vi "Read_IMU.vi"(6 "error in (no error) 2":errorcluster, 8 "IMU_SS":T1, 9 "SPI Ref In":T8={"myRIO Reference"={"myRIO Model"=enum."Unknown", "myRIO Hardware Reference"={"Generic FPGA Reference"=refnum, "Allow multiple opens"=FALSE}}, "SPI Channels Enum"=enum."Not Connected", "SPI Configuration"={"Frequency [Hz]"=0.0, "Clock Phase"=enum."Leading", "Clock Polarity"=enum."Low", "Data Direction"=enum."Most significant bit first", "Frame Length"=8}} {"SPI Configuration"."Frame Length" min=1 max=16}) -> (0 "error out":errorcluster, 1 "Roll":dbl, 2 "Yaw":dbl, 3 "Pitch":dbl)   [LabVIEW 2018]
uses:
  <vilib>/myRIO/Instrument Drivers/Onboard IO/SPI/typedefs/SPI Reference.ctl
  <vilib>/myRIO/Common/Instrument Driver Framework/Utilities/typedefs/myRIO Generic Hardware Reference.ctl
  <vilib>/myRIO/Common/Instrument Driver Framework/Utilities/typedefs/Hardware Version Enum.ctl
  <vilib>/myRIO/Common/Instrument Driver Framework/Utilities/typedefs/myRIO v1.0 Reference.ctl
  <vilib>/myRIO/Common/Instrument Driver Framework/Utilities/typedefs/Generic FPGA Reference.ctl
  <vilib>/myRIO/Common/Instrument Driver Framework/myRIO v1.0/SPI/typedefs/SPI Channels Enum.ctl
  <vilib>/myRIO/Instrument Drivers/Onboard IO/SPI/typedefs/SPI Configuration.ctl
  <vilib>/myRIO/Common/Instrument Driver Framework/myRIO v1.0/SPI/typedefs/SPI Clock Phase.ctl
  <vilib>/myRIO/Common/Instrument Driver Framework/myRIO v1.0/SPI/typedefs/SPI Clock Polarity.ctl
  <vilib>/myRIO/Common/Instrument Driver Framework/myRIO v1.0/SPI/typedefs/SPI Data Direction.ctl
  <vilib>/myRIO/Common/Instrument Driver Framework/myRIO v1.0/SPI/typedefs/SPI Frame Length.ctl
  <vilib>/myRIO/Instrument Drivers/Onboard IO/DIO/typedefs/DIO Reference.ctl
  <vilib>/myRIO/Common/Instrument Driver Framework/myRIO v1.0/DIO/typedefs/DIO Channels List.ctl
  <vilib>/myRIO/Common/Instrument Driver Framework/myRIO v1.0/DIO/typedefs/DIO Channels Enum.ctl
  <vilib>/Utility/error.llb/Error Cluster From Error Code.vi
  <vilib>/myRIO/Common/Instrument Driver Framework/myRIO v1.0/DIO/vis/myRIO v1.0 Write DIO.vi
  <vilib>/myRIO/Common/Instrument Driver Framework/myRIO v1.0/SPI/vis/myRIO v1.0 Write Read SPI.vi
  <vilib>/myRIO/Instrument Drivers/Onboard IO/SPI/SPI.lvlib
  <vilib>/myRIO/Instrument Drivers/Onboard IO/DIO/DIO.lvlib
panel:
  out "subarray":u16[](array[numeric])
  out "IMU":sgl[](array[numeric])
  out "IMU_SS":T1
  out "SPI Ref Out":T8={"myRIO Reference"={"myRIO Model"=enum."Unknown", "myRIO Hardware Reference"={"Generic FPGA Reference"=refnum, "Allow multiple opens"=FALSE}}, "SPI Channels Enum"=enum."Not Connected", "SPI Configuration"={"Frequency [Hz]"=0.0, "Clock Phase"=enum."Leading", "Clock Polarity"=enum."Low", "Data Direction"=enum."Most significant bit first", "Frame Length"=8}} {"SPI Configuration"."Frame Length" min=1 max=16}
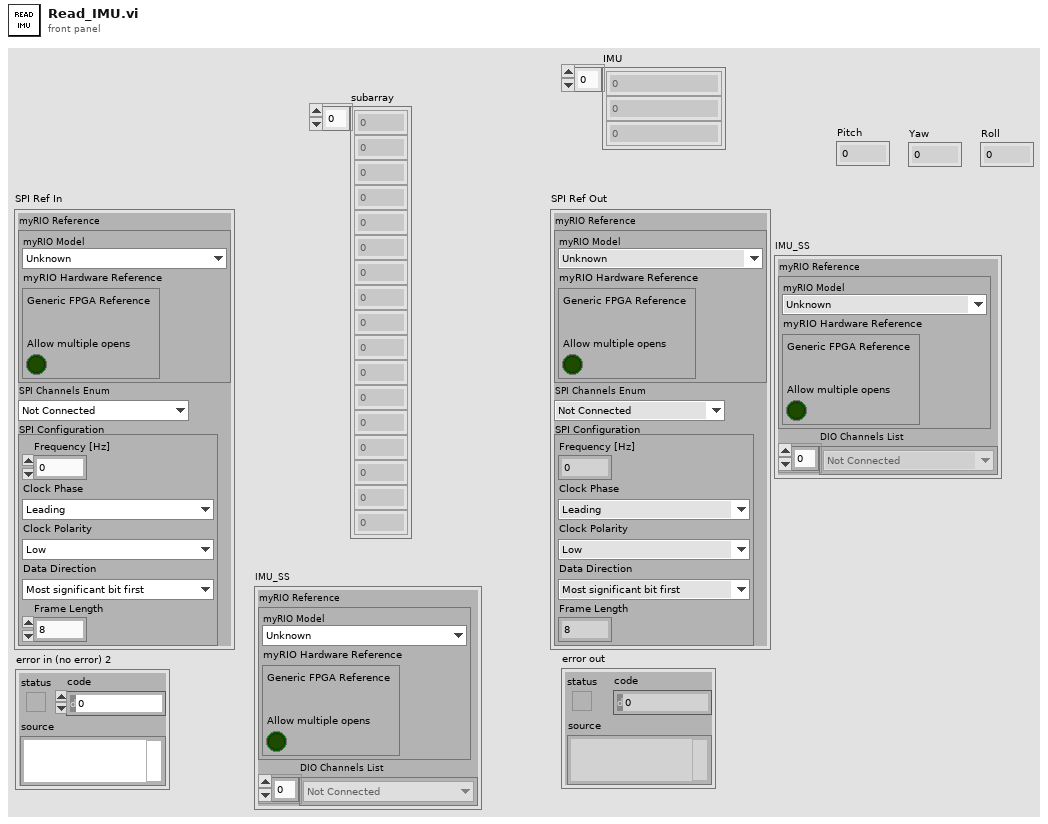
[diagram p1: front panel]
types:
  T1 = typedef "DIO.lvlib/DIO Reference.ctl" = cluster{"myRIO Reference":T2, "DIO Channels List":T6}
  T2 = typedef "myRIO Generic Hardware Reference.ctl" = cluster{"myRIO Model":T3, "myRIO Hardware Reference":T4}
  T3 = typedef "Hardware Version Enum.ctl" = enum16{"Unknown", "myRIO-1900", "myRIO-1950", "roboRIO", "NI ELVIS RIO CM", "ELVIS III"}
  T4 = typedef "myRIO v1.0 Reference.ctl" = cluster{"Generic FPGA Reference":T5, "Allow multiple opens":bool}
  T5 = typedef "Generic FPGA Reference.ctl" = refnum<k20>
  T6 = typedef "DIO Channels List.ctl" = T7[]
  T7 = typedef "DIO Channels Enum.ctl" = enum16{"Not Connected", "C/DIO0", "C/DIO1", "C/DIO2", "C/DIO3", "C/DIO4", "C/DIO5", "C/DIO6", "C/DIO7", "A/DIO0", "A/DIO1", "A/DIO2", "A/DIO3", "A/DIO4", "A/DIO5", "A/DIO6", "A/DIO7", "A/DIO8", "A/DIO9", "A/DIO10", "A/DIO11", "A/DIO12", "A/DIO13", "A/DIO14", "A/DIO15", "A/DIO16", "A/DIO17", "A/DIO18", "A/DIO19", "B/DIO0", "B/DIO1", "B/DIO2", "B/DIO3", "B/DIO4", "B/DIO5", "B/DIO6", "B/DIO7", "B/DIO8", "B/DIO9", "B/DIO10", "B/DIO11", "B/DIO12", "B/DIO13", "B/DIO14", "B/DIO15", "B/DIO16", "B/DIO17", "B/DIO18", "B/DIO19", "LED0", "LED1", "LED2", "LED3", "Button0", "DIO/DIO0", "DIO/DIO1", "DIO/DIO2", "DIO/DIO3", "DIO/DIO4", "DIO/DIO5", "DIO/DIO6", "DIO/DIO7", "DIO/DIO8", "DIO/DIO9", "SPI/CS0", "SPI/CS1", "SPI/CS2", "SPI/CS3", "LED RADIO (Green)", "LED RADIO (Red)", "LED COMM (Green)", "LED COMM (Red)", "LED MODE (Green)", "LED MODE (Red)"}
  T8 = typedef "SPI.lvlib/SPI Reference.ctl" = cluster{"myRIO Reference":T2, "SPI Channels Enum":T9, "SPI Configuration":T10}
  T9 = typedef "SPI Channels Enum.ctl" = enum16{"Not Connected", "A/SPI", "B/SPI", "SPI/SPI"}
  T10 = typedef "SPI.lvlib/SPI Configuration.ctl" = cluster{"Frequency [Hz]":dbl, "Clock Phase":T11, "Clock Polarity":T12, "Data Direction":T13, "Frame Length":T14}
  T11 = typedef "SPI Clock Phase.ctl" = enum8{"Leading", "Trailing"}
  T12 = typedef "SPI Clock Polarity.ctl" = enum8{"Low", "High"}
  T13 = typedef "SPI Data Direction.ctl" = enum8{"Most significant bit first", "Least significant bit first"}
  T14 = typedef "SPI Frame Length.ctl" = u8
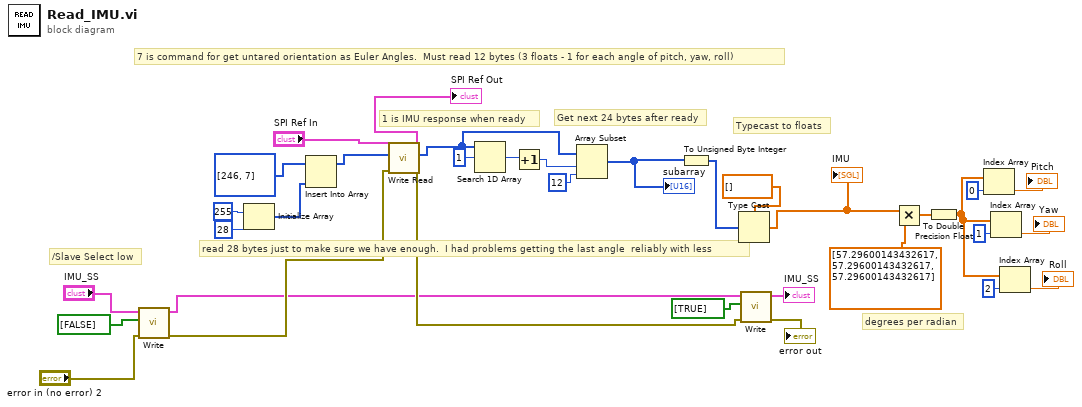
[diagram p0: block diagram]
diagram:
  # "degrees per radian"
  # "read 28 bytes just to make sure we have enough.  I had problems getting the last angle  reliably with less"
  # "/Slave Select low"
  # "Typecast to floats"
  # "Get next 24 bytes after ready"
  # "1 is IMU response when ready"
  # "7 is command for get untared orientation as Euler Angles.  Must read 12 bytes (3 floats - 1 for each angle of pitch, yaw, roll)"
  n1 = call <vilib>:"Write.vi"("error in (no error)"="error in (no error) 2", "Values"=bool[] [FALSE], "DIO Ref In"="IMU_SS") -> ("error out"=w16:errorcluster, "DIO Ref Out"=w14:T1)  [unwired: 6 in]
  n2 = Initialize Array(u16 255 ("element"), 28 ("dimension size")) -> (w20:u16[])
  n3 = Insert Into Array(array=u16[] [246, 7] ("Frames to Write"), new element=w20) -> (w29:u16[])  [unwired: 1 in]
  n4 = call <vilib>:"Write Read.vi"("error in (no error)"=w16, "Frames to Write"=w29, "SPI Ref In"="SPI Ref In") -> ("error out"=w15:errorcluster, "Frames Read"=w22:u16[], "SPI Ref Out"=→"SPI Ref Out":T8)  [unwired: 6 in]
  n5 = Search 1D Array(1D array=w22, element=u16 1) -> (index of element=w27:i32)  [unwired: 1 in]
  n6 = Increment(x=w27) -> (x+1=w26:i32)
  n7 = Array Subset(array=w22, index=w26, length=12) -> (w24:u16[])
  "subarray" <- w24
  n8 = To Unsigned Byte Integer(number=w24) -> (unsigned 8bit integer=w33:u8[])
  n9 = Type Cast(type=sgl[] [], x=w33) -> (*(type *) &x=w10:sgl[])
  "IMU" <- w10
  n10 = call <vilib>:"Write.vi"("error in (no error)"=w15, "Values"=bool[] [TRUE], "DIO Ref In"=w14) -> ("error out"=→"error out":errorcluster, "DIO Ref Out"=→"IMU_SS":T1)  [unwired: 6 in]
  n11 = Multiply(x=w10, y=sgl[] [57.296, 57.296, 57.296]) -> (x*y=w8:sgl[])
  n12 = To Double Precision Float(number=w8) -> (double precision float=w1:dbl[])
  n13 = Index Array(array=w1, index=0) -> (element=→"Pitch":dbl)
  n14 = Index Array(array=w1, index=1) -> (element=→"Yaw":dbl)
  n15 = Index Array(array=w1, index=2) -> (element=→"Roll":dbl)
